vi "Change AcroField Value (String).vi"(0 "PDF Path (original)":path, 2 "FormFlattening":bool, 5 "PDF Path (modified )":path, 7 "AcroField Name":string, 9 "AcroField Value":string, 11 "error in (no error)":errorcluster, 13 "Owner Password":string) -> (4 "File Name":path, 15 "error out":errorcluster)   [LabVIEW 2020, in "Exaprom PDF.lvlib"]
doc: "BSD License (http://www.opensource.org/licenses/)\n\nCopyright© 2013, Exaprom Inc\nAll rights reserved."
uses:
  <userlib>/labview-PDF-writer-master/Exaprom PDF.lvlib
  <userlib>/labview-PDF-writer-master/Controls/Initialization Controls/File Permission Parameters.ctl
  C:/Program Files (x86)/National Instruments/LabVIEW 2020/user.lib/labview-PDF-writer-master/DLL/itextsharp.dll
  DLL/itextsharp.dll
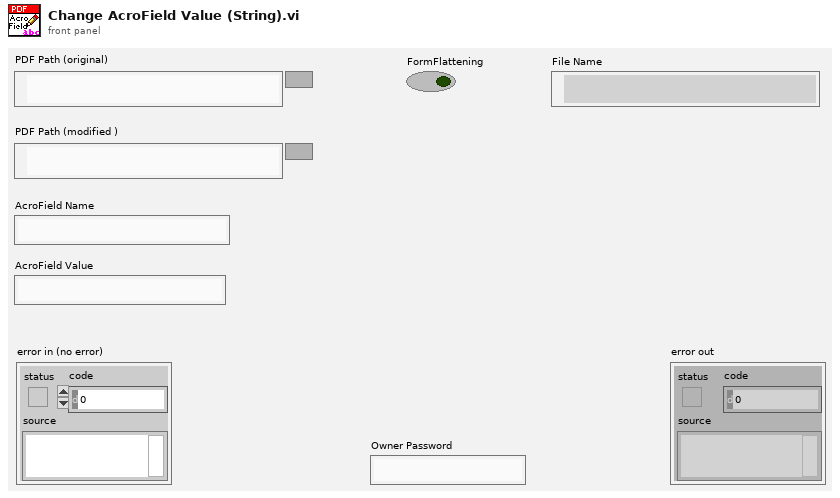
[diagram p1: front panel]
types:
  T1 = typedef "Exaprom PDF.lvlib/File Permission Parameters.ctl" = cluster{"User Password":string, "Owner Password":string, "Printing":enum16{"Allow Printing", "Allow Degraded Printing", "Don't Allow Printing"}, "Allow Modify Contents":bool, "Allow Copy":bool, "Allow Modify Annotations":bool, "Allow Fill In ":bool, "Allow Screen Readers":bool, "Allow Assembly":bool}
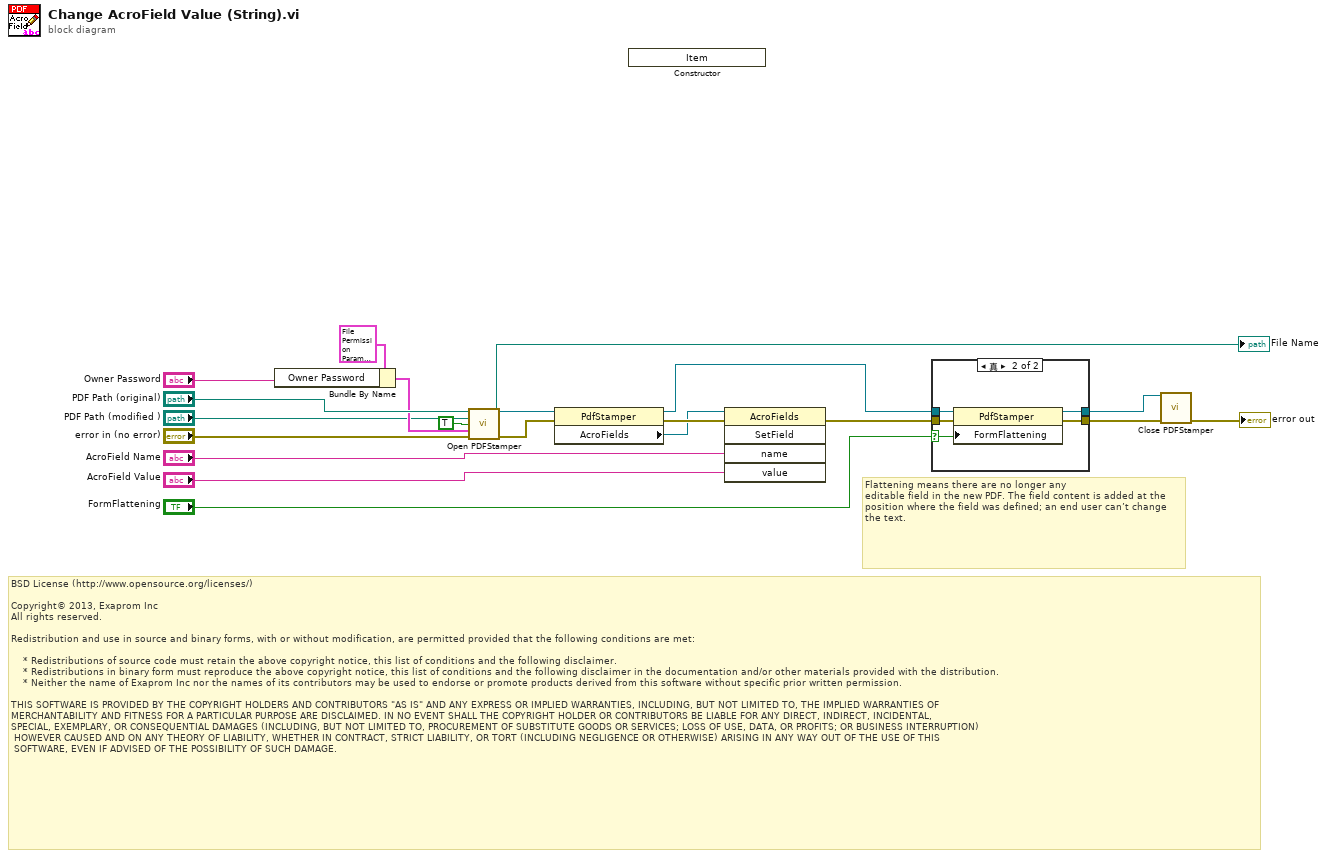
[diagram p0: block diagram]
diagram:
  # "BSD License (http://www.opensource.org/licenses/)\n\nCopyright© 2013, Exaprom Inc\nAll rights reserved.\n\nRedistribution and use in source and binary forms, with or without modification, are permitted provided that the following conditions are met:\n\n    * Redistributions of source code must retain the above copyright notice, this list of conditions and the following disclaimer.\n    * Redistributions in binary form must reproduce the above copyright notice, this list of conditions and the following disclaimer in the documentation and/or other materials provided with the distribution.\n    * Neither the name of Exaprom Inc nor the names of its contributors may be used to endorse or promote products derived from this software without specific prior written permission.\n\nTHIS SOFTWARE IS PROVIDED BY THE COPYRIGHT HOLDERS AND CONTRIBUTORS \"AS IS\" AND ANY EXPRESS OR IMPLIED WARRANTIES, INCLUDING, BUT NOT LIMITED TO, THE IMPLIED WARRANTIES OF \nMERCHANTABILITY AND FITNESS FOR A PARTICULAR PURPOSE ARE DISCLAIMED. IN NO EVENT SHALL THE COPYRIGHT HOLDER OR CONTRIBUTORS BE LIABLE FOR ANY DIRECT, INDIRECT, INCIDENTAL,\nSPECIAL, EXEMPLARY, OR CONSEQUENTIAL DAMAGES (INCLUDING, BUT NOT LIMITED TO, PROCUREMENT OF SUBSTITUTE GOODS OR SERVICES; LOSS OF USE, DATA, OR PROFITS; OR BUSINESS INTERRUPTION)\n HOWEVER CAUSED AND ON ANY THEORY OF LIABILITY, WHETHER IN CONTRACT, STRICT LIABILITY, OR TORT (INCLUDING NEGLIGENCE OR OTHERWISE) ARISING IN ANY WAY OUT OF THE USE OF THIS\n SOFTWARE, EVEN IF ADVISED OF THE POSSIBILITY OF SUCH DAMAGE."
  # "Flattening means there are no longer any\neditable field in the new PDF. The field content is added at the position where the field was defined; an end user can’t change the text."
  n1 = Bundle By Name(cluster=T1 {"User Password"="", "Owner Password"="", "Printing"=enum."Allow Printing", "Allow Modify Contents"=FALSE, "Allow Copy"=FALSE, "Allow Modify Annotations"=TRUE, "Allow Fill In "=TRUE, "Allow Screen Readers"=FALSE, "Allow Assembly"=FALSE} ("Permissions"), "Owner Password"="Owner Password") -> (w3:T1)
  n2 = call <userlib>:"Open PDFStamper.vi"("PDF Path (original)"="PDF Path (original)", "PDF Path (modified )"="PDF Path (modified )", "RotateContents (F)"=TRUE, "Permissions"=w3, "error in (no error)"="error in (no error)") -> ("PDFStamper"=w17:refnum<k24>, "Temporary File Name"=→"File Name":path, "error out"=w15:errorcluster)  [unwired: 2 in, 6 out]
  n3 = property class="PdfStamper"(reference=w17, error in=w15) -> (reference out=w16:refnum<k24>, error out=w14:errorcluster, "AcroFields"=w1:refnum<k24>)
  n4 = constructor class="AcroFields+Item"() -> ()  [unwired: 3 in, 3 out]
  n5 = invoke class="AcroFields" method="SetField"(reference=w1, error in=w14, "name"="AcroField Name", "value"="AcroField Value") -> (error out=w13:errorcluster)  [unwired: 1 in, 4 out]
  n6 = case shown="真" "FormFlattening" {
    selector: "FormFlattening" -> [_ w23]
    tunnel: w16 -> [w21 w27]
    tunnel: w13 -> [w22 w26]
    tunnel: [w22 w25] -> w12
    tunnel: [w21 w24] -> w11
    frame False {
    }
    frame True {
      n7 = property class="PdfStamper"(reference=w27, error in=w26, "FormFlattening"=w23) -> (reference out=w24:refnum<k24>, error out=w25:errorcluster)
    }
  }
  n8 = call <userlib>:"Close PDFStamper.vi"("PDFStamper"=w11, "error in (no error)"=w12) -> ("error out"=→"error out":errorcluster)  [unwired: 13 in]
